vi "Conditum Entity Editor.vi"   [LabVIEW 2020]
uses:
  Conditum-Tools/Entity Editor/Entity Editor.lvclass
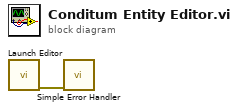
[diagram p0: block diagram]
diagram:
  n1 = call "Launch Editor.vi"() -> ("error out"=w1:errorcluster)  [unwired: 11 in]
  n2 = call <vilib>:"Simple Error Handler.vi"("error in (no error)"=w1) -> ()  [unwired: 4 in, 5 out]
